vi "remote-reg.vi"(7 "Enum":enum16{"read", "write"}(ring), 10 "write":T1) -> (2 "read":T1)   [LabVIEW 2019]
uses:
  ctl/remote.ctl
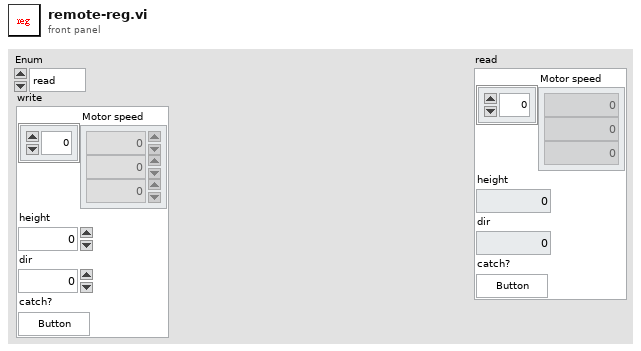
[diagram p1: front panel]
types:
  T1 = typedef "remote.ctl" = cluster{"Motor speed":dbl[], "height":dbl, "dir":i32, "catch?":bool}
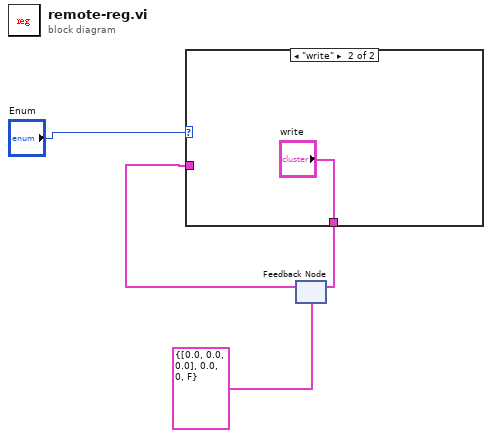
[diagram p0: block diagram]
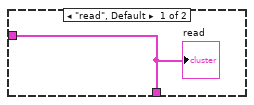
[diagram p2: hidden frame]
diagram:
  n1 = feedback #1(T1 {"Motor speed"=[0.0, 0.0, 0.0], "height"=0.0, "dir"=0, "catch?"=FALSE} ("Cluster")) -> (w2:T1)
  n2 = case shown="\"write\"" "Enum" {
    tunnel: w2 -> [w5 _]
    tunnel: [w5 "write"] -> w1
    frame "read", Default {
      "read" <- w5
    }
    frame "write" {
    }
  }
  n3 = feedback-in #1(w1) -> ()
